vi "Hausmodell.ParameterUI.vi"() -> ()   [LabVIEW 2016, in "Hausmodell.lvclass"]
uses:
  Hausmodell.lvclass
  Package ResourceControl/ViHandler/ViHandler.ViInfo.ctl
  Package Libraries/Message Queue/private/MessageQueue.MessageTypeDef.ctl
  Hausmodell.lvclass/Hausmodell.ctl
  Package ErrorHandling/ErrorHandling.lvclass/ErrorHandling.ctl
  Read Parameter.Hausmodell.vi
  Package ErrorHandling/ErrorHandling.checkForErrorAndHandle.vi
  Package ErrorHandling/ErrorHandling.GetErrorHandler.vi
  Package Libraries/StringFunctions/StringFunctions_ReplaceAllBlindSigns.vi
  <vilib>/dlg_ctls.llb/Space Constant.vi
  <vilib>/Utility/error.llb/Error Cluster From Error Code.vi
  Package Libraries/TimingFunctions/TimingFunctions_getUtcTimestamp.vi
  <vilib>/Utility/error.llb/Trim Whitespace.vi
  <vilib>/Utility/error.llb/Search and Replace Pattern.vi
  Package ErrorHandling/ErrorHandling.addLastErrorToFile.vi
  <vilib>/ErrorRing/Error Ring.xnode
  Package ErrorHandling/ErrorHandling.lvclass
  Package ResourceControl/ViHandler/ViHandler.lvclass
panel:
  in  "Hausmodell Parameter":T1={"Bodenfläche [m2]"=4000.0, "Raumhöhe [m]"=1.2, "Bodendicke [m]"=0.05, "Hausmaterial Dichte [kg/m3]"=0.0, "Hausmaterial Spez. Wärmekapazität [J/KgK]"=0.0, "U-Wert Boden [W/m2/K]"=0.0, "U-Wert Fenster [W/m2K]"=0.0, "U-Wert Wand/Dach [W/m2K]"=0.0, "Heizrohr Aussenradius [m]"=0.0, "Heizrohr Innenradius [m]"=0.0, "Heizrohr Wärmeleitfähigkeit [W/mK]"=0.0, "Heizrohr Länge pro m2 Bodenfläche [m] "=0.0, "Heizwasser Volumenstrom [m3/h]"=0.0, "Heizwasser Dichte [Kg/m3]"=0.0, "Heizwasser Spez. Wärmekapazität [J/KgK]"=0.0} {"Heizwasser Spez. Wärmekapazität [J/KgK]" min=0.0 max=10000.0 format="%#.0f"; "Heizwasser Dichte [Kg/m3]" min=0.0 max=10000.0 format="%#.0f"; "Heizwasser Volumenstrom [m3/h]" min=0.0 max=50.0 format="%#.1f"; "Heizrohr Länge pro m2 Bodenfläche [m]" min=0.0 max=10.0 format="%#.1f"; "Heizrohr Wärmeleitfähigkeit [W/mK]" min=0.0 max=100.0 format="%#.2f"; "Heizrohr Innenradius [m]" min=0.0 max=0.1 format="%#.3f"; "Heizrohr Aussenradius [m]" min=0.0 max=0.1 format="%#.3f"; "U-Wert Wand/Dach [W/m2K]" min=0.0 max=20.0 format="%#.2f"; "U-Wert Fenster [W/m2K]" min=0.0 max=20.0 format="%#.2f"; "U-Wert Boden [W/m2/K]" min=0.0 max=20.0 format="%#.2f"; "Hausmaterial Spez. Wärmekapazität [J/KgK]" min=0.0 max=10000.0 format="%#.0f"; "Hausmaterial Dichte [kg/m3]" min=0.0 max=10000.0 format="%#.0f"; "Bodendicke [m]" min=0.05 max=0.5 format="%#.2f"; "Raumhöhe [m]" min=1.0 max=5.0 format="%#.0f"; "Bodenfläche [m2]" min=0.0 max=6000.0 format="%#.0f"}
  in  "Model Path":path
  out "Hausmodell":refnum<data-value>
  out "ViInfoTemp":T2
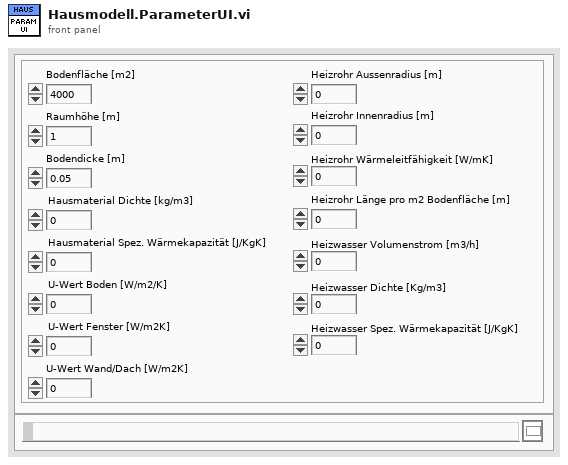
[diagram p1: front panel]
types:
  T1 = cluster{"Bodenfläche [m2]":dbl, "Raumhöhe [m]":dbl, "Bodendicke [m]":dbl, "Hausmaterial Dichte [kg/m3]":dbl, "Hausmaterial Spez. Wärmekapazität [J/KgK]":dbl, "U-Wert Boden [W/m2/K]":dbl, "U-Wert Fenster [W/m2K]":dbl, "U-Wert Wand/Dach [W/m2K]":dbl, "Heizrohr Aussenradius [m]":dbl, "Heizrohr Innenradius [m]":dbl, "Heizrohr Wärmeleitfähigkeit [W/mK]":dbl, "Heizrohr Länge pro m2 Bodenfläche [m] ":dbl, "Heizwasser Volumenstrom [m3/h]":dbl, "Heizwasser Dichte [Kg/m3]":dbl, "Heizwasser Spez. Wärmekapazität [J/KgK]":dbl}
  T2 = typedef "ViHandler.lvclass/ViHandler.ViInfo.ctl" = cluster{"ViName":string, "ViReference":refnum<vi>, "ViQueueName":string}
  T3 = typedef "MessageQueue.MessageTypeDef.ctl" = cluster{"Message":string, "Data":variant}
  T4 = enum16{"open", "replace", "create", "open or create", "replace or create", "replace or create with confirmation"}
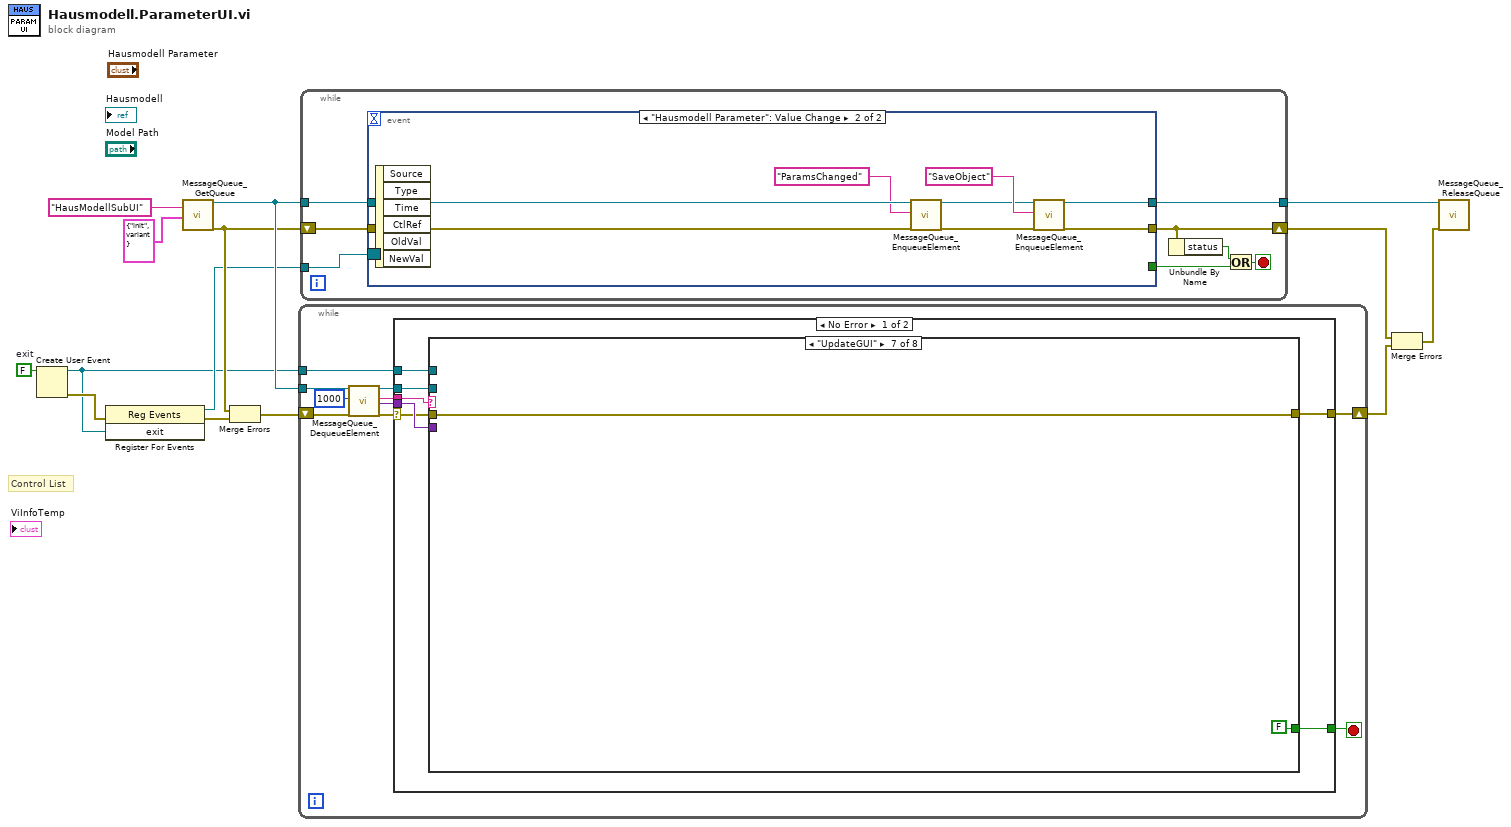
[diagram p0: block diagram]
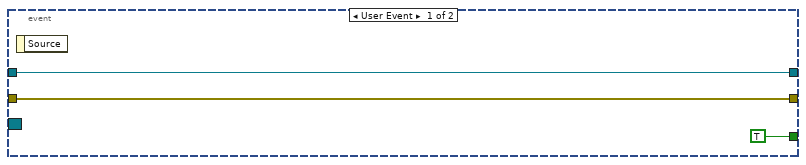
[diagram p2: hidden frame]
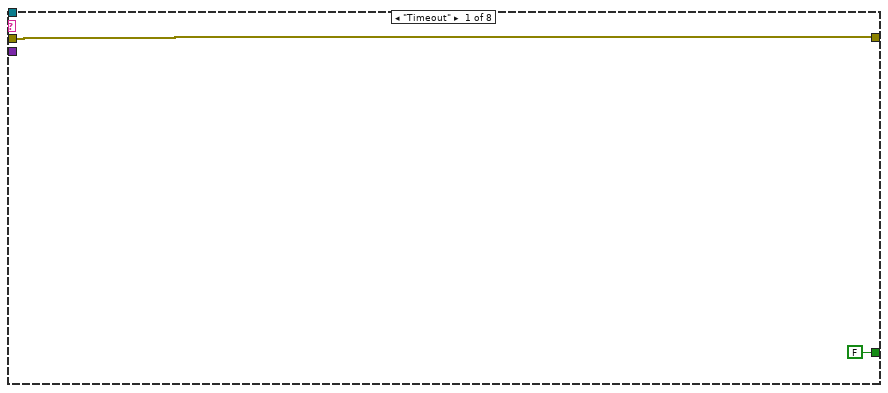
[diagram p3: hidden frame]
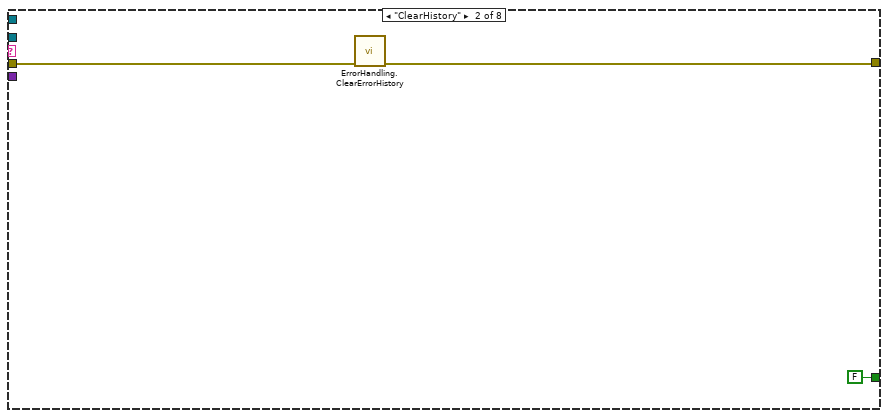
[diagram p4: hidden frame]
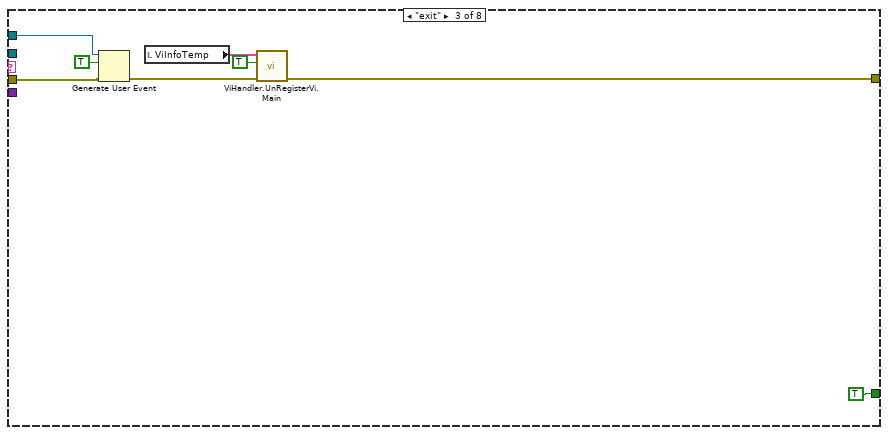
[diagram p5: hidden frame]
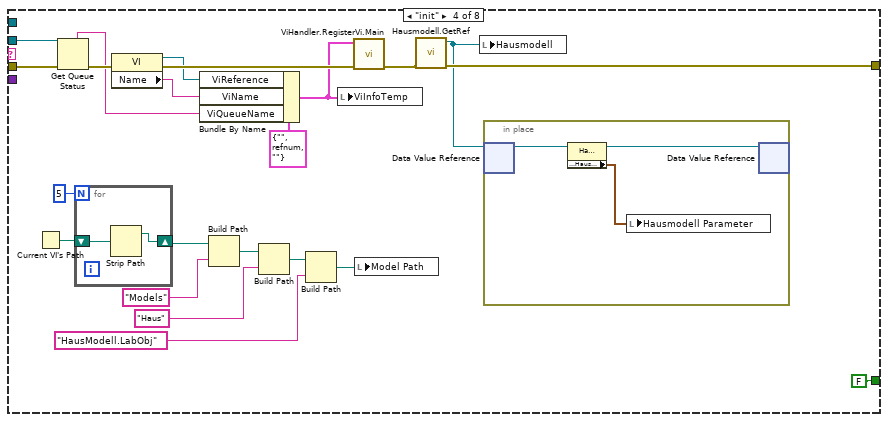
[diagram p6: hidden frame]
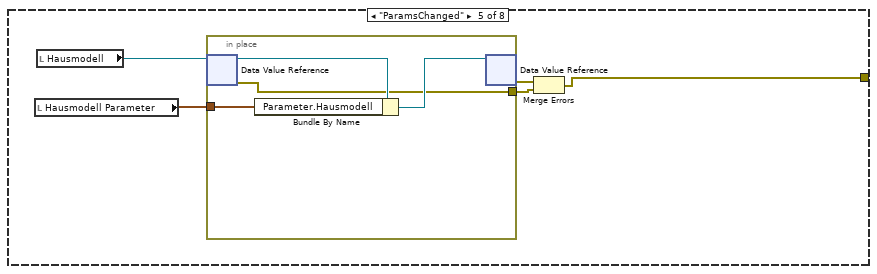
[diagram p7: hidden frame]
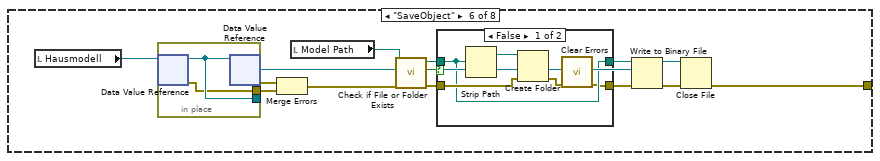
[diagram p8: hidden frame]
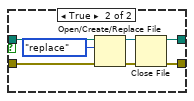
[diagram p9: hidden frame]
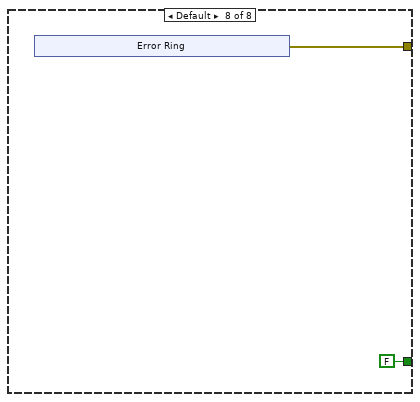
[diagram p10: hidden frame]
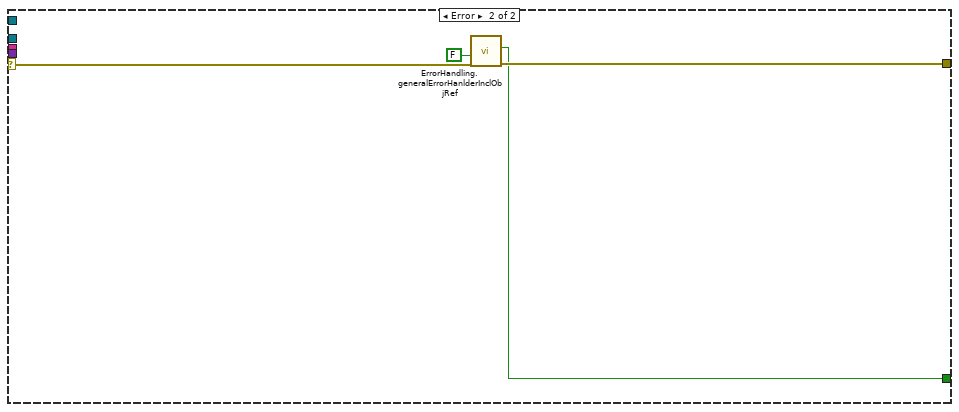
[diagram p11: hidden frame]
diagram:
  w7 = FALSE  # exit
  # "Control List"
  n1 = Create User Event(user event datatype=w7) -> (user event=w5:refnum<user-event>, error out=w6:errorcluster)  [unwired: 1 in]
  n2 = register-events(error in=w6, w5) -> (reference out=w9:refnum<event-registration>, error out=w11:errorcluster)  [unwired: 1 in]
  n3 = call "MessageQueue_GetQueue.vi"("Name"="HausModellSubUI", "OptionalInitValue"=T3 {"Message"="init", "Data"=variant}) -> ("QueueOut"=w13:refnum<queue>, "ErrorOut"=w10:errorcluster)  [unwired: 15 in, 1 out]
  n4 = Merge Errors(w10, w11) -> (w8:errorcluster)
  n5 = while {
    tunnel: w13 -> [w24]
    tunnel: w5 -> [w17]
    shift-right: [w16] -> w3
    shift-left: w8 -> [w18]
    stop <- w19 stop-if-true
    n6 = call "MessageQueue_DequeueElement.vi"("QueueIn"=w24, "Timeout"=1000, "ErrorIn"=w18) -> ("QueueOut"=w22:refnum<queue>, "Message"=w21:string, "Data"=w20:variant, "ErrorOut"=w23:errorcluster)  [unwired: 12 in, 1 out]
    n7 = case shown="No Error" w23 {
      selector: w23 -> [w27 w121]
      tunnel: w22 -> [w31 _]
      tunnel: w21 -> [w30 _]
      tunnel: w20 -> [w29 _]
      tunnel: [w28 w119] -> w19
      tunnel: w17 -> [w26 _]
      tunnel: [w25 w120] -> w16
      frame No Error {
        n8 = case shown="\"UpdateGUI\"" w30 {
          tunnel: w31 -> [_ _ _ w60 _ _ _ _]
          tunnel: w29 -> [_ _ _ _ _ _ _ _]
          tunnel: [FALSE FALSE TRUE FALSE _ _ FALSE FALSE] -> w28
          tunnel: w27 -> [w32 w35 w42 w57 _ _ w109 _]
          tunnel: w26 -> [_ _ w41 _ _ _ _ _]
          tunnel: [w32 w34 w38 w55 w72 w82 w109 w112] -> w25
          frame "Timeout" {
          }
          frame "ClearHistory" {
            n9 = call "ErrorHandling.ClearErrorHistory.vi"("error IO"=w35) -> ("error IO"=w34:errorcluster)  [unwired: 10 in]
          }
          frame "exit" {
            n10 = Generate User Event(user event=w41, event data cluster=TRUE ("event data"), error in=w42) -> (error out=w39:errorcluster)  [unwired: 1 in, 1 out]
            n11 = local read "ViInfoTemp"() -> (w40:T2)
            n12 = call "ViHandler.UnRegisterVi.Main.vi"("ErrorIn"=w39, "FinalExit?"=TRUE, "ViInfo"=w40) -> ("ErrorOut"=w38:errorcluster)  [unwired: 7 in, 1 out]
          }
          frame "init" {
            n13 = Current VI's Path() -> (path=w46:path)
            n14 = Get Queue Status(queue=w60, error in (no error)=w57) -> (queue name=w58:string, error out=w64:errorcluster)  [unwired: 1 in, 6 out]
            n15 = for {
              N: 5 -> [_]
              shift-right: [w67] -> w52
              shift-left: w46 -> [w68]
              n16 = Strip Path(path=w68) -> (stripped path=w67:path)  [unwired: 1 out]
            }
            n17 = property class="VI"(error in=w64) -> (reference out=w62:refnum<vi>, error out=w63:errorcluster, "Name"=w61:string)  [unwired: 1 in]
            n18 = Bundle By Name(cluster=T2 {"ViName"="", "ViReference"=refnum, "ViQueueName"=""} ("ViInfo"), "ViReference"=w62, "ViName"=w61, "ViQueueName"=w58) -> (w59:T2)
            n19 = Build Path(base path=w52, name or relative path="Models") -> (appended path=w50:path)
            n20 = Build Path(base path=w50, name or relative path="Haus") -> (appended path=w48:path)
            n21 = Build Path(base path=w48, name or relative path="HausModell.LabObj") -> (appended path=w45:path)
            n22 = local write "ViInfoTemp"(w59) -> ()
            n23 = call "ViHandler.RegisterVi.Main.vi"("ErrorIn"=w63, "ViInfo"=w59) -> ("ErrorOut"=w56:errorcluster)  [unwired: 9 in]
            n24 = local write "Model Path"(w45) -> ()
            n25 = call "Hausmodell.GetRef.vi"("Error In"=w56) -> ("Error out"=w55:errorcluster, "Hausmodell"=w54:refnum<data-value>)  [unwired: 9 in]
            n26 = local write "Hausmodell"(w54) -> ()
            n27 = in-place {
              n28 = in-place-dvr #1(w54) -> (w71:refnum<class "Hausmodell.lvclass">)  [unwired: 1 out]
              n29 = property class="Hausmodell.lvclass"(reference=w71) -> (reference out=w70:refnum<class "Hausmodell.lvclass">, "Accessors:Parameter.Hausmodell"=w69:T1)  [unwired: 1 in, 1 out]
              n30 = local write "Hausmodell Parameter"(w69) -> ()
              n31 = in-place-dvr #1(w70) -> ()  [unwired: 2 out]
            }
          }
          frame "ParamsChanged" {
            n32 = local read "Hausmodell Parameter"() -> (w75:T1)
            n33 = local read "Hausmodell"() -> (w76:refnum<data-value>)
            n34 = in-place {
              in-place-border: w75 -> [w78]
              in-place-border: [w77] -> w73
              n35 = in-place-dvr #2(w76) -> (w80:refnum<class "Hausmodell.lvclass">, w77:errorcluster)
              n36 = Bundle By Name(cluster=w80, "Parameter.Hausmodell"=w78) -> (w79:refnum<class "Hausmodell.lvclass">)
              n37 = in-place-dvr #2(w79) -> (w74:errorcluster)  [unwired: 1 out]
            }
            n38 = Merge Errors(w74, w73) -> (w72:errorcluster)
          }
          frame "SaveObject" {
            n39 = local read "Hausmodell"() -> (w94:refnum<data-value>)
            n40 = in-place {
              in-place-border: [w108] -> w88
              in-place-border: [w107] -> w86
              n41 = in-place-dvr #3(w94) -> (w108:refnum<class "Hausmodell.lvclass">, w107:errorcluster)
              n42 = in-place-dvr #3(w108) -> (w87:errorcluster)  [unwired: 1 out]
            }
            n43 = Merge Errors(w87, w86) -> (w85:errorcluster)
            n44 = local read "Model Path"() -> (w81:path)
            n45 = call <vilib>:"Check if File or Folder Exists.vi"("error in (no error)"=w85, "path"=w81) -> ("error out"=w91:errorcluster, "file or folder exists?"=w93:bool, "dup path"=w92:path)  [unwired: 7 in]
            n46 = case shown="False" w93 {
              tunnel: w92 -> [w97 w106]
              tunnel: [w97 w102] -> w90
              tunnel: w91 -> [w98 w105]
              tunnel: [w95 w101] -> w89
              frame False {
                n47 = Strip Path(path=w97) -> (stripped path=w99:path)  [unwired: 1 out]
                n48 = Create Folder(path (use dialog)=w99, error in=w98) -> (error out=w96:errorcluster)  [unwired: 1 in, 2 out]
                n49 = call <vilib>:"Clear Errors.vi"("error in (no error)"=w96) -> ("error out"=w95:errorcluster)  [unwired: 5 in, 1 out]
              }
              frame True {
                n50 = Open/Create/Replace File(file path (use dialog)=w106, error in=w105, operation (0:open)=T4."replace") -> (refnum out=w103:refnum<file>, error out=w100:errorcluster)  [unwired: 3 in, 1 out]
                n51 = Close File(refnum=w103, error in=w100) -> (path=w102:path, error out=w101:errorcluster)
              }
            }
            n52 = Write to Binary File(file (use dialog)=w90, data=w88, error in=w89) -> (refnum out=w83:refnum<file>, error out=w84:errorcluster)  [unwired: 3 in, 1 out]
            n53 = Close File(refnum=w83, error in=w84) -> (error out=w82:errorcluster)  [unwired: 1 out]
          }
          frame "UpdateGUI" {
          }
          frame Default {
            n54 = xnode "Error Ring"() -> ("error out"=w112:errorcluster)
          }
        }
      }
      frame Error {
        n55 = call "ErrorHandling.generalErrorHanlderInclObjRef.vi"("error in"=w121, "StopOnError"=FALSE) -> ("error out"=w120:errorcluster, "Stop"=w119:bool)  [unwired: 7 in, 1 out]
      }
    }
  }
  n56 = while {
    tunnel: w13 -> [w129]
    tunnel: [w128] -> w14
    shift-right: [w125] -> w2
    shift-left: w10 -> [w127]
    tunnel: w9 -> [w122]
    stop <- w124 stop-if-true
    n57 = event shown="[1] \"Hausmodell Parameter\": Value Change" {
      selector: w122 -> [_ _]
      dyn-events: _ -> [_ _]
      timeout: _ -> [_ _]
      tunnel: w129 -> [w131 w140]
      tunnel: [w131 w134] -> w128
      tunnel: [w130 w133] -> w125
      tunnel: w127 -> [w130 w139]
      tunnel: [TRUE _] -> w126
      event User Event {
        n58 = event-data() -> ()  [unwired: 1 in, 1 out]
      }
      event "Hausmodell Parameter": Value Change {
        n59 = event-data() -> ()  [unwired: 1 in, 6 out]
        n60 = call "MessageQueue_EnqueueElement.vi"("QueueIn"=w140, "Message"="ParamsChanged", "ErrorIn"=w139) -> ("QueueOut"=w136:refnum<queue>, "ErrorOut"=w135:errorcluster)  [unwired: 15 in]
        n61 = call "MessageQueue_EnqueueElement.vi"("QueueIn"=w136, "Message"="SaveObject", "ErrorIn"=w135) -> ("QueueOut"=w134:refnum<queue>, "ErrorOut"=w133:errorcluster)  [unwired: 15 in]
      }
    }
    n62 = Unbundle By Name(w125) -> ("status"=w123:bool)
    n63 = Or(x=w123, y=w126) -> (x .or. y?=w124:bool)
  }
  n64 = Merge Errors(w2, w3) -> (w1:errorcluster)
  n65 = call "MessageQueue_ReleaseQueue.vi"("QueueIn"=w14, "ErrorIn"=w1) -> ()  [unwired: 15 in, 3 out]
